vi "usrp set tx antenna.vi"(8 "error in (no error)":errorcluster, 9 "chan":u64, 10 "ant":string, 11 "h":u64) -> (0 "error out":errorcluster, 2 "function return":u32(ring), 3 "h 2":u64)   [LabVIEW 2024, in "uhd.lvlib"]
doc: "UHD_API uhd_error uhd_usrp_set_tx_antenna(\n uhd_usrp_handle h, const char* ant, size_t chan);"
uses:
  uhd.lvlib
  uhd.so
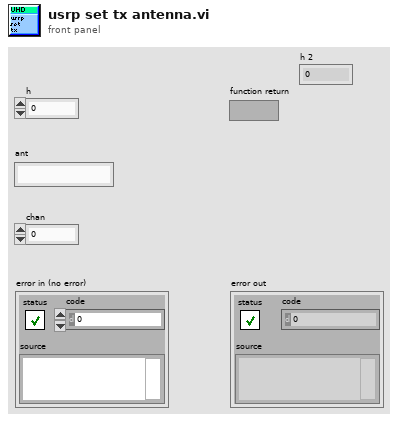
[diagram p1: front panel]
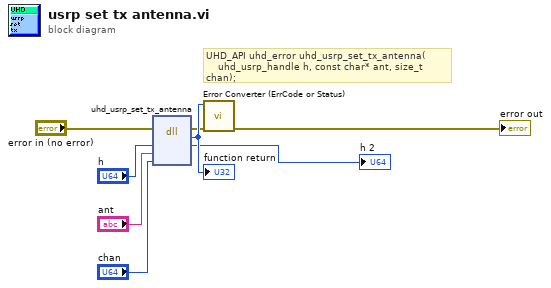
[diagram p0: block diagram]
diagram:
  # "UHD_API uhd_error uhd_usrp_set_tx_antenna(\n    uhd_usrp_handle h, const char* ant, size_t chan);"
  n1 = dll-call lib="uhd.*" fn="uhd_usrp_set_tx_antenna"(error in="error in (no error)", "h"="h", "ant"="ant", "chan"="chan") -> (error out=w3:errorcluster, w8:u32, "h"=→"h 2":u64)  [unwired: 4 in, 1 out]
  "function return" <- w8
  n2 = call "Error Converter (ErrCode or Status).vi"("error in (no error)"=w3, "error code"=w8) -> ("error out"=→"error out":errorcluster)  [unwired: 9 in]
